vi "executeLastCommand.vi"(8 "error in (no error)":errorcluster, 11 "Monochromator in":refnum<class "Monochromator.lvclass">) -> (0 "error out":errorcluster, 3 "Monochromator out":refnum<class "Monochromator.lvclass">)   [LabVIEW 2016, in "Monochromator.lvclass"]
uses:
  Monochromator.lvclass
  Monochromator.lvclass/Monochromator.ctl
  Commands/Command/Command.lvclass
  Commands/CommandQueue/CommandQueue.lvclass
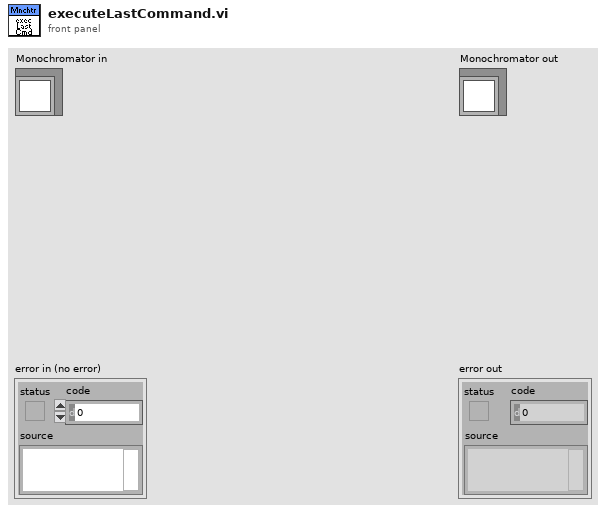
[diagram p1: front panel]
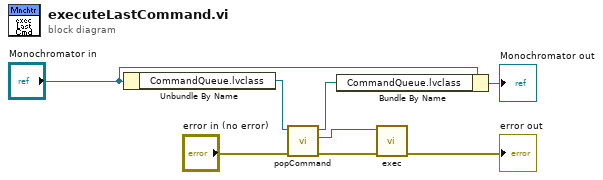
[diagram p0: block diagram]
diagram:
  n1 = Unbundle By Name("Monochromator in") -> ("CommandQueue.lvclass"=w5:refnum<class "CommandQueue.lvclass">)
  n2 = call "popCommand.vi"("error in (no error)"="error in (no error)", "CommandQueue in"=w5) -> ("error out"=w3:errorcluster, "Command"=w4:refnum<class "Command.lvclass">, "CommandQueue out"=w2:refnum<class "CommandQueue.lvclass">)  [unwired: 7 in]
  n3 = Bundle By Name(cluster="Monochromator in", "CommandQueue.lvclass"=w2) -> (→"Monochromator out":refnum<class "Monochromator.lvclass">)
  n4 = call-dynamic "exec.vi"("error in (no error)"=w3, "Command in"=w4) -> ("error out"=→"error out":errorcluster)  [unwired: 8 in, 1 out]
